vi "DWDT Uncompress Digital.vi"(8 "error in (no error)":errorcluster, 11 "compressed digital waveform":digitalwaveform(waveform)={"t0"=timestamp(0 s since 1904-01-01), "dt"=0.0, "Y"={"transitions"=[], "data"=[]}, "error"={"status"=FALSE, "code"=37421928, "source"=""}}) -> (0 "error out":errorcluster, 3 "uncompressed digital waveform":digitalwaveform(waveform)={"t0"=timestamp(0 s since 1904-01-01), "dt"=0.0, "Y"={"transitions"=[], "data"=[]}, "error"={"status"=FALSE, "code"=37421928, "source"=""}})   [LabVIEW 2011]
doc: "Uncompresses the digital signals in the digital input and returns the result in the digital output. Wire data to the <B>uncompressed digital waveform</B> input to determine the polymorphic instance to use or manually select the instance."
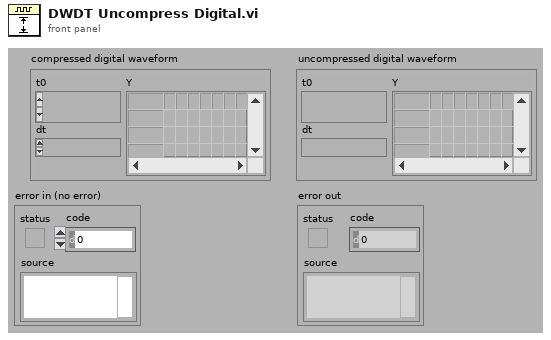
[diagram p1: front panel]
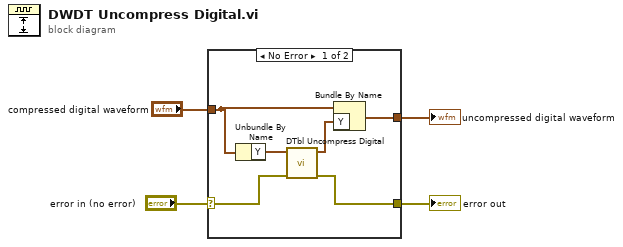
[diagram p0: block diagram]
diagram:
  n1 = case shown="No Error" "error in (no error)" {
    selector: "error in (no error)" -> [w6 w12]
    tunnel: [w7 w11] -> w4
    tunnel: "compressed digital waveform" -> [w9 w11]
    tunnel: [w5 w12] -> w1
    frame No Error {
      n2 = Unbundle By Name(w9) -> ("Y"=w10:digitaldata)
      n3 = call "DTbl Uncompress Digital.vi"("error in (no error)"=w6, "digital data in"=w10) -> ("error out"=w5:errorcluster, "digital data out"=w8:digitaldata)  [unwired: 8 in]
      n4 = Bundle By Name(cluster=w9, "Y"=w8) -> (w7:digitalwaveform)
    }
    frame Error {
    }
  }
  "uncompressed digital waveform" <- w4
  "error out" <- w1
